vi "PhotonTrackedTarget_Equals.vi"(9 "Other TrackedTarget":T1={"Yaw"=0.0, "Pitch"=0.0, "Area"=0.0, "Skew"=0.0, "MinAreaRectCorners"=[], "BestCameraToTarget"={"TRANSLATION3D"={"X"=0.0, "Y"=0.0, "Z"=0.0}, "ROTATION3D"={"Q_quaternion"={"R"=1.0, "V"=[0.0, 0.0, 0.0]}}, "XF"=FALSE}, "FiducialId"=0, "AltCameraToTarget"={"TRANSLATION3D"={"X"=0.0, "Y"=0.0, "Z"=0.0}, "ROTATION3D"={"Q_quaternion"={"R"=1.0, "V"=[0.0, 0.0, 0.0]}}, "XF"=FALSE}, "PoseAmbiguity"=0.0, "DetectedCorners"=[], "ObjDetectId"=0, "ObjDetectConf"=0.0} {"AltCameraToTarget"."TRANSLATION3D"."Z" format="%14.3f"; "AltCameraToTarget"."TRANSLATION3D"."Y" format="%14.3f"; "AltCameraToTarget"."TRANSLATION3D"."X" format="%14.3f"; "BestCameraToTarget"."TRANSLATION3D"."Z" format="%14.3f"; "BestCameraToTarget"."TRANSLATION3D"."Y" format="%14.3f"; "BestCameraToTarget"."TRANSLATION3D"."X" format="%14.3f"}, 11 "TrackedTarget":T1={"Yaw"=0.0, "Pitch"=0.0, "Area"=0.0, "Skew"=0.0, "MinAreaRectCorners"=[], "BestCameraToTarget"={"TRANSLATION3D"={"X"=0.0, "Y"=0.0, "Z"=0.0}, "ROTATION3D"={"Q_quaternion"={"R"=1.0, "V"=[0.0, 0.0, 0.0]}}, "XF"=FALSE}, "FiducialId"=0, "AltCameraToTarget"={"TRANSLATION3D"={"X"=0.0, "Y"=0.0, "Z"=0.0}, "ROTATION3D"={"Q_quaternion"={"R"=1.0, "V"=[0.0, 0.0, 0.0]}}, "XF"=FALSE}, "PoseAmbiguity"=0.0, "DetectedCorners"=[], "ObjDetectId"=0, "ObjDetectConf"=0.0} {"AltCameraToTarget"."TRANSLATION3D"."Z" format="%14.3f"; "AltCameraToTarget"."TRANSLATION3D"."Y" format="%14.3f"; "AltCameraToTarget"."TRANSLATION3D"."X" format="%14.3f"; "BestCameraToTarget"."TRANSLATION3D"."Z" format="%14.3f"; "BestCameraToTarget"."TRANSLATION3D"."Y" format="%14.3f"; "BestCameraToTarget"."TRANSLATION3D"."X" format="%14.3f"}) -> (3 "Equals":bool)   [LabVIEW 2019, in "PhotonVisionLib.lvlib"]
doc: "Determines if two tracked targets are equal\n\nInputs:\n - TrackedTarget -- TrackedTarget cluster.\n - OtherTrackedTarget -- Second TrackedTarget cluster.\n\nOutputs:\n - Area -- Boolean, equals TRUE if both TrackedTargets are the same."
uses:
  PhotonVisionLib.lvlib
  TypeDef/PhotonTrackedTargetType.ctl
  TypeDef/TargetCornerType.ctl
  <vilib>/Rock Robotics/WPI/ThirdParty/JAS_Junk/TrajLib/TypeDef/TRANSFORM3D.ctl
  <vilib>/Rock Robotics/WPI/ThirdParty/JAS_Junk/TrajLib/TypeDef/TRANSLATION3D.ctl
  <vilib>/Rock Robotics/WPI/ThirdParty/JAS_Junk/TrajLib/TypeDef/ROTATION3D.ctl
  <vilib>/Rock Robotics/WPI/ThirdParty/JAS_Junk/TrajLib/TypeDef/QUATERNION.ctl
  <vilib>/Rock Robotics/WPI/ThirdParty/JAS_Junk/TrajLib/VI/Transform3d_GetTranslation3d.vi
  <vilib>/Rock Robotics/WPI/ThirdParty/JAS_Junk/TrajLib/VI/Transform3d_GetRotation3d.vi
  <vilib>/Rock Robotics/WPI/ThirdParty/JAS_Junk/TrajLib/VI/Rotation3d_Equals.vi
  <vilib>/Rock Robotics/WPI/ThirdParty/JAS_Junk/TrajLib/VI/Translation3d_Equals.vi
  <vilib>/Rock Robotics/WPI/ThirdParty/JAS_Junk/TrajLib/VI/Rotation3d_GetQuaterion.vi
  <vilib>/Rock Robotics/WPI/ThirdParty/JAS_Junk/TrajLib/VI/Quaternion_Equals.vi
  <vilib>/Rock Robotics/WPI/ThirdParty/JAS_Junk/TrajLib/VI/Quaternion_Get_Vect.vi
  <vilib>/Rock Robotics/WPI/ThirdParty/JAS_Junk/TrajLib/VI/Quaternion_Get_W.vi
  <vilib>/Rock Robotics/WPI/ThirdParty/JAS_Junk/TrajLib/Trajectory_Library.lvlib
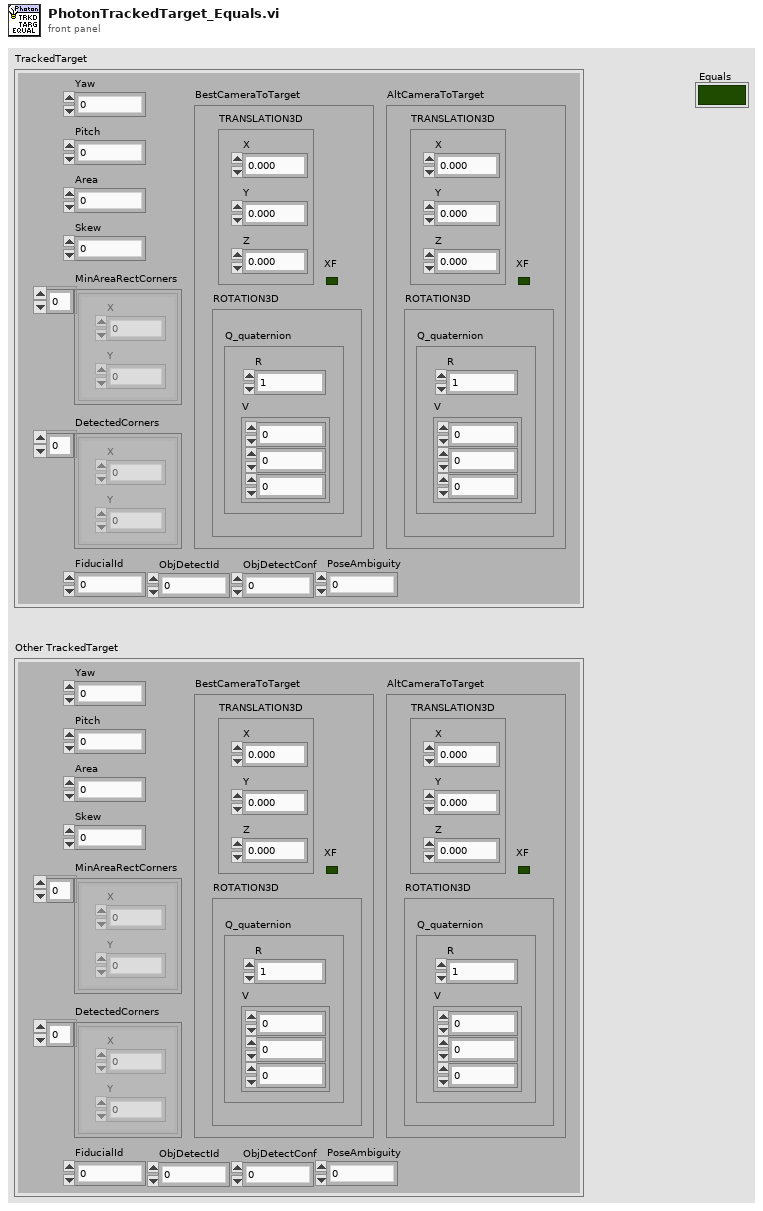
[diagram p1: front panel]
types:
  T1 = typedef "PhotonVisionLib.lvlib/PhotonTrackedTargetType.ctl" = cluster{"Yaw":dbl, "Pitch":dbl, "Area":dbl, "Skew":dbl, "MinAreaRectCorners":T2[], "BestCameraToTarget":T3, "FiducialId":i32, "AltCameraToTarget":T3, "PoseAmbiguity":dbl, "DetectedCorners":T2[], "ObjDetectId":i32, "ObjDetectConf":sgl}
  T2 = typedef "PhotonVisionLib.lvlib/TargetCornerType.ctl" = cluster{"X":dbl, "Y":dbl}
  T3 = typedef "Trajectory_Library.lvlib/TRANSFORM3D.ctl" = cluster{"TRANSLATION3D":T4, "ROTATION3D":T5, "XF":bool}
  T4 = typedef "Trajectory_Library.lvlib/TRANSLATION3D.ctl" = cluster{"X":dbl, "Y":dbl, "Z":dbl}
  T5 = typedef "Trajectory_Library.lvlib/ROTATION3D.ctl" = cluster{"Q_quaternion":T6}
  T6 = typedef "Trajectory_Library.lvlib/QUATERNION.ctl" = cluster{"R":dbl, "V":dbl[]}
  T7 = cluster{"Yaw":bool, "Pitch":bool, "Area":bool, "Skew":bool, "MinAreaRectCorners":cluster{"X":bool, "Y":bool}[], "BestCameraToTarget":cluster{"TRANSLATION3D":cluster{"X":bool, "Y":bool, "Z":bool}, "ROTATION3D":cluster{"Q_quaternion":cluster{"R":bool, "V":bool[]}}, "XF":bool}, "FiducialId":bool, "AltCameraToTarget":cluster{"TRANSLATION3D":cluster{"X":bool, "Y":bool, "Z":bool}, "ROTATION3D":cluster{"Q_quaternion":cluster{"R":bool, "V":bool[]}}, "XF":bool}, "PoseAmbiguity":bool, "DetectedCorners":cluster{"X":bool, "Y":bool}[], "ObjDetectId":bool, "ObjDetectConf":bool}
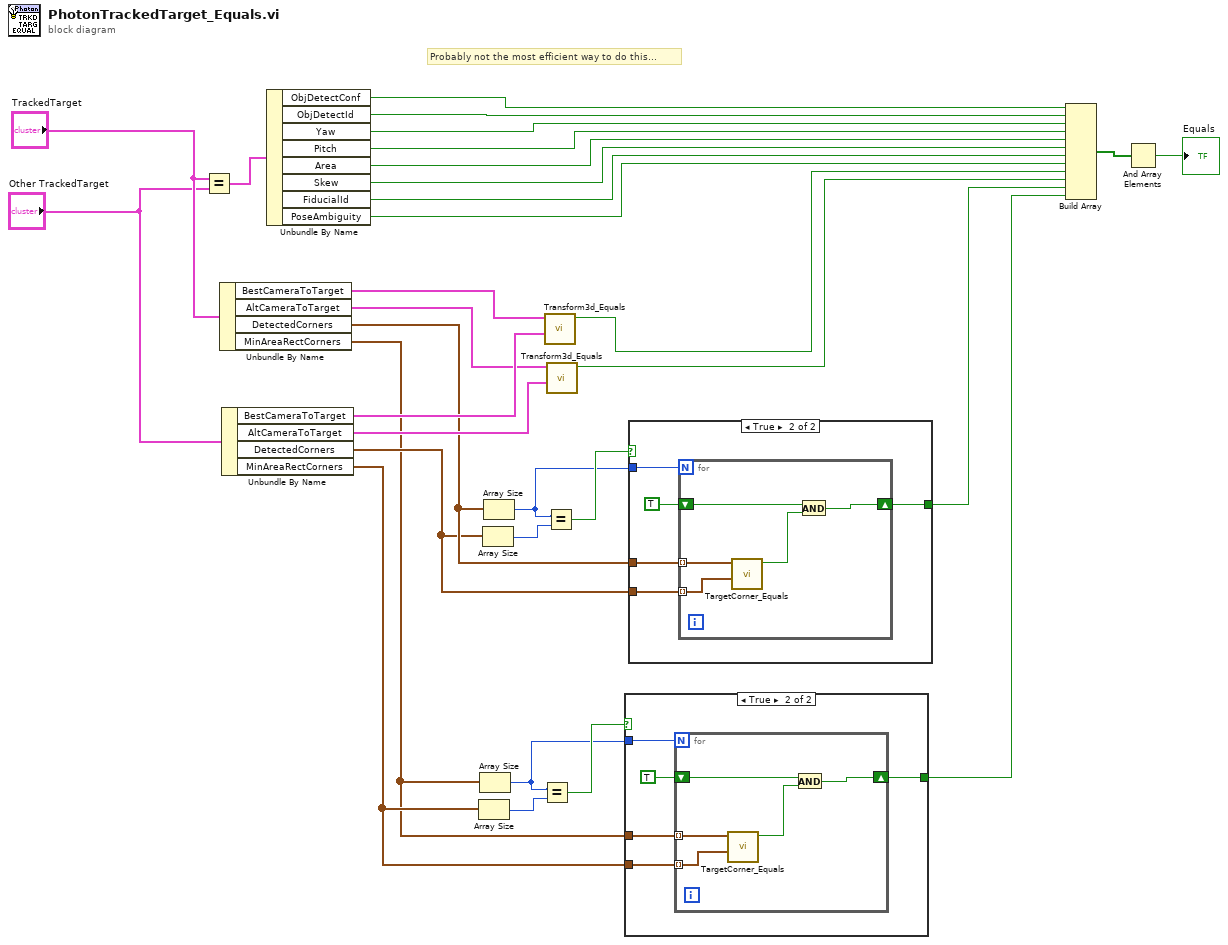
[diagram p0: block diagram]
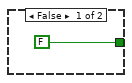
[diagram p2: hidden frame]
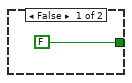
[diagram p3: hidden frame]
diagram:
  # "Probably not the most efficient way to do this..."
  n1 = Equal?(x="TrackedTarget", y="Other TrackedTarget") -> (x = y?=w31:T7)
  n2 = Unbundle By Name("TrackedTarget") -> ("BestCameraToTarget"=w20:T3, "AltCameraToTarget"=w18:T3, "DetectedCorners"=w11:T2[], "MinAreaRectCorners"=w4:T2[])
  n3 = Unbundle By Name("Other TrackedTarget") -> ("BestCameraToTarget"=w19:T3, "AltCameraToTarget"=w17:T3, "DetectedCorners"=w10:T2[], "MinAreaRectCorners"=w5:T2[])
  n4 = Unbundle By Name(w31) -> ("ObjDetectConf"=w1:bool, "ObjDetectId"=w2:bool, "Yaw"=w30:bool, "Pitch"=w29:bool, "Area"=w28:bool, "Skew"=w27:bool, "FiducialId"=w26:bool, "PoseAmbiguity"=w25:bool)
  n5 = Array Size(array=w5) -> (size(s)=w8:i32)
  n6 = Array Size(array=w4) -> (size(s)=w6:i32)
  n7 = Array Size(array=w10) -> (size(s)=w14:i32)
  n8 = Array Size(array=w11) -> (size(s)=w12:i32)
  n9 = Equal?(x=w6, y=w8) -> (x = y?=w7:bool)
  n10 = call <vilib>:"Transform3d_Equals.vi"("otherTransform3d"=w19, "inTransform3d"=w20) -> ("Equals"=w16:bool)  [unwired: 9 in]
  n11 = Equal?(x=w12, y=w14) -> (x = y?=w13:bool)
  n12 = call <vilib>:"Transform3d_Equals.vi"("otherTransform3d"=w17, "inTransform3d"=w18) -> ("Equals"=w15:bool)  [unwired: 9 in]
  n13 = case shown="True" w7 {
    tunnel: [FALSE w33] -> w3
    tunnel: w6 -> [_ w36]
    tunnel: w4 -> [_ w35]
    tunnel: w5 -> [_ w34]
    frame False {
    }
    frame True {
      n14 = for {
        N: w36 -> [_]
        shift-right: [w41] -> w33
        shift-left: TRUE -> [w42]
        tunnel: w35 -> [w40] mode=indexing
        tunnel: w34 -> [w39] mode=indexing
        n15 = call "TargetCorner_Equals.vi"("Other TargetCorner"=w39, "TargetCorner"=w40) -> ("Equals"=w38:bool)  [unwired: 9 in]
        n16 = And(x=w42, y=w38) -> (x .and. y?=w41:bool)
      }
    }
  }
  n17 = case shown="True" w13 {
    tunnel: [FALSE w44] -> w9
    tunnel: w12 -> [_ w47]
    tunnel: w11 -> [_ w46]
    tunnel: w10 -> [_ w45]
    frame False {
    }
    frame True {
      n18 = for {
        N: w47 -> [_]
        shift-right: [w52] -> w44
        shift-left: TRUE -> [w53]
        tunnel: w46 -> [w51] mode=indexing
        tunnel: w45 -> [w50] mode=indexing
        n19 = call "TargetCorner_Equals.vi"("Other TargetCorner"=w50, "TargetCorner"=w51) -> ("Equals"=w49:bool)  [unwired: 9 in]
        n20 = And(x=w53, y=w49) -> (x .and. y?=w52:bool)
      }
    }
  }
  n21 = Build Array(w1, w2, w30, w29, w28, w27, w26, w25, w16, w15, w9, w3) -> (w24:bool[])
  n22 = And Array Elements(Boolean array=w24) -> (logical AND=→"Equals":bool)
